vi "create_full_request_data.vi"(0 "llm_anthropic_chatmodels in":refnum<class "llm_anthropic_chatmodels.lvclass">, 5 "Messages":refnum<class "abstract_message_base.lvclass">[](array[class]), 11 "error in (no error)":errorcluster) -> (4 "llm_anthropic_chatmodels out":refnum<class "llm_anthropic_chatmodels.lvclass">, 6 "Request Data":string, 15 "error out":errorcluster)   [LabVIEW 2020, in "llm_anthropic_chatmodels.lvclass"]
uses:
  llm_anthropic_chatmodels.lvclass
  D:/Personal/LabVIEW LLMs/src/models/abstract_llm_base/abstract_llm_base.lvclass
  abstract_message_base/abstract_message_base.lvclass
  utils/anthropic_chatmodel_request_data.ctl
  llm_anthropic_chatmodels.lvclass/llm_anthropic_chatmodels.ctl
  message_text/message_text.lvclass
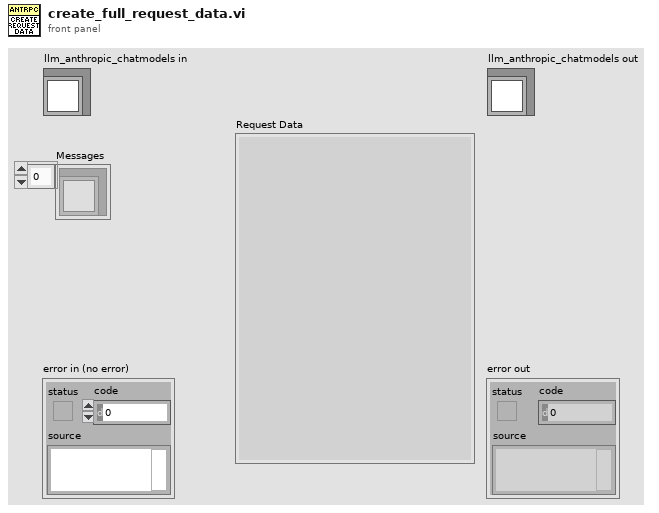
[diagram p1: front panel]
types:
  T1 = typedef "llm_anthropic_chatmodels.lvclass/anthropic_chatmodel_request_data.ctl" = cluster{"model":string, "messages":cluster{"role":string, "content":cluster{"type":string, "text":string}[]}[], "temperature":dbl, "max_tokens":u32, "top_p":dbl, "system":string}
  T2 = typedef "message_text.lvclass/message.ctl" = cluster{"role":string, "content":string[]}
  T3 = cluster{"role":string, "content":cluster{"type":string, "text":string}[]}
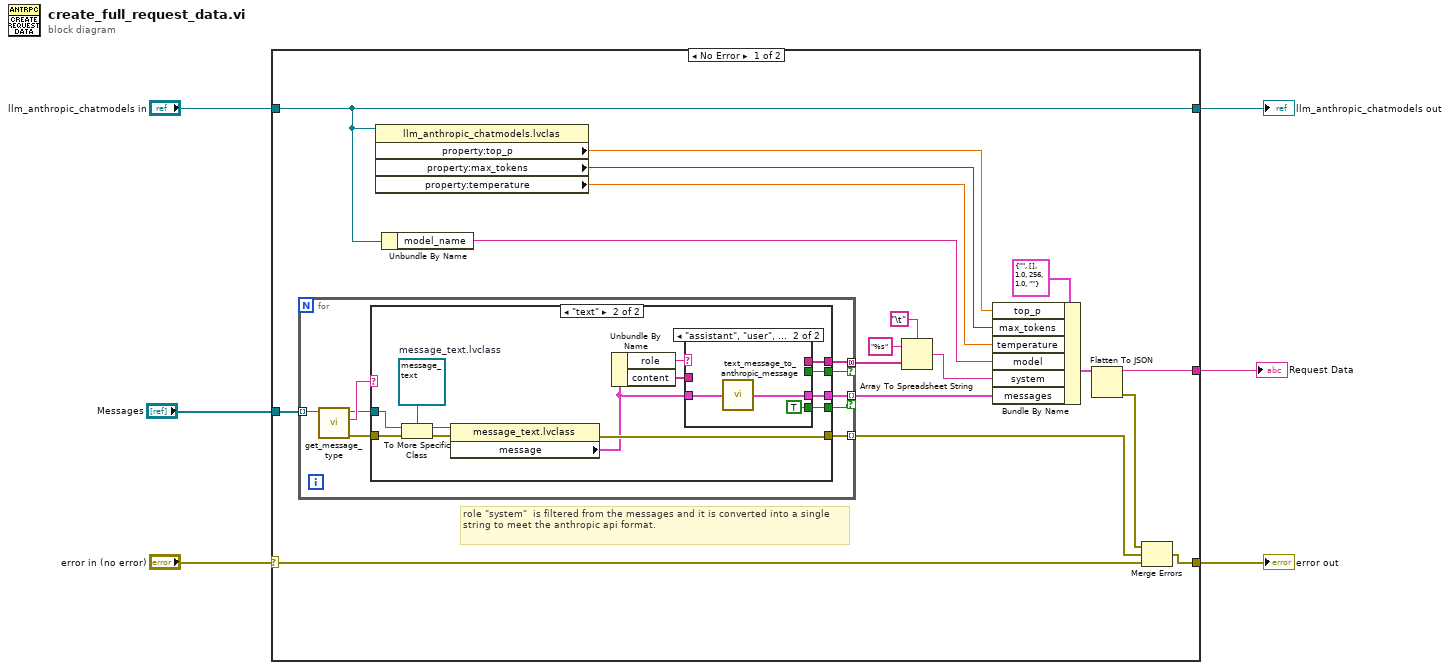
[diagram p0: block diagram]
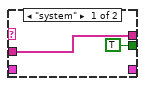
[diagram p3: hidden frame]
diagram:
  n1 = case shown="No Error" "error in (no error)" {
    selector: "error in (no error)" -> [w24 w54]
    tunnel: [w19 w54] -> w5
    tunnel: [w15 w53] -> w3
    tunnel: "llm_anthropic_chatmodels in" -> [w15 w53]
    tunnel: "Messages" -> [w22 _]
    tunnel: [w16 _] -> w1
    frame No Error {
      # "role \"system\"  is filtered from the messages and it is converted into a single string to meet the anthropic api format."
      n2 = for {
        tunnel: w22 -> [w33] mode=indexing
        tunnel: [w29] -> w18 mode=indexing
        tunnel: [w28] -> w21 mode=indexing if=w25
        tunnel: [w27] -> w10 mode=concatenating if=w26
        n3 = call-dynamic "get_message_type.vi"("abstract_message_base in"=w33) -> ("error out"=w30:errorcluster, "Type"=w32:string, "abstract_message_base out"=w31:refnum<class "abstract_message_base.lvclass">)  [unwired: 8 in]
        n4 = case shown="\"text\"" w32 {
          tunnel: w31 -> [_ w46]
          tunnel: w30 -> [w34 w47]
          tunnel: [w34 w42] -> w29
          tunnel: [_ w41] -> w28
          tunnel: [_ w38] -> w27
          tunnel: [_ w36] -> w26
          tunnel: [_ w35] -> w25
          frame Default {
          }
          frame "text" {
            w45 = refnum<class "message_text.lvclass"> refnum  # message_text.lvclass
            n5 = To More Specific Class(target class=w45, reference=w46, error in=w47) -> (specific class reference=w44:refnum<class "message_text.lvclass">, error out=w43:errorcluster)
            n6 = property class="message_text.lvclass"(reference=w44, error in=w43) -> (error out=w42:errorcluster, "message"=w40:T2)  [unwired: 1 out]
            n7 = Unbundle By Name(w40) -> ("role"=w39:string, "content"=w37:string[])
            n8 = case shown="\"assistant\", \"user\", Default" w39 {
              tunnel: [_ w52] -> w41
              tunnel: w40 -> [_ w51]
              tunnel: [w49 _] -> w38
              tunnel: w37 -> [w49 _]
              tunnel: [TRUE _] -> w36
              tunnel: [_ TRUE] -> w35
              frame "system" {
              }
              frame "assistant", "user", Default {
                n9 = call "text_message_to_anthropic_message.vi"("message"=w51) -> ("message out"=w52:T3)
              }
            }
          }
        }
      }
      n10 = property class="llm_anthropic_chatmodels.lvclas"(reference=w15) -> ("property:top_p"=w14:dbl, "property:max_tokens"=w13:u32, "property:temperature"=w12:dbl)  [unwired: 1 in, 2 out]
      n11 = Unbundle By Name(w15) -> ("model_name"=w11:string)
      n12 = Array To Spreadsheet String(delimiter (Tab)="\t", array=w10, 3:"%s" ("format string")) -> (spreadsheet string=w8:string)
      n13 = Bundle By Name(cluster=T1 {"model"="", "messages"=[], "temperature"=1.0, "max_tokens"=256, "top_p"=1.0, "system"=""} ("data"), "top_p"=w14, "max_tokens"=w13, "temperature"=w12, "model"=w11, "system"=w8, "messages"=w21) -> (w20:T1)
      n14 = Flatten To JSON(anything=w20) -> (JSON string=w16:string, 11:w17:errorcluster)  [unwired: 2 in]
      n15 = Merge Errors(w17, w18, w24) -> (w19:errorcluster)
    }
    frame Error {
    }
  }
  "error out" <- w5
  "llm_anthropic_chatmodels out" <- w3
  "Request Data" <- w1
